vi "DFD M-Band Filter Bank Decomposition (Array).vi"(7 "init? (F)":bool, 8 "error in (no error)":errorcluster, 10 "filter bank in":T1 {"mFBank_SynthesisFilters"."mMRate_SumWl" min=1 max=32 step=1; "mFBank_SynthesisFilters"."mMRate_InputIwl" min=1 max=32 step=1; "mFBank_SynthesisFilters"."mMRate_GainWl" min=1 max=32 step=1; "mFBank_SynthesisFilters"."mMRate_OutputWl" min=1 max=32 step=1; "mFBank_SynthesisFilters"."mMRate_InputWl" min=1 max=32 step=1; "mFBank_SynthesisFilters"."mMRate_CoefWl" min=1 max=32 step=1; "mFBank_SynthesisFilters"."mMRate_Mode" items=["Default"=-1, "No Rate Change"=0, "Interpolation"=1, "Decimation"=2, "Interpolated"=3, "Rational"=4]; "mFBank_AnalysisFilters"."mMRate_SumWl" min=1 max=32 step=1; "mFBank_AnalysisFilters"."mMRate_InputIwl" min=1 max=32 step=1; "mFBank_AnalysisFilters"."mMRate_GainWl" min=1 max=32 step=1; "mFBank_AnalysisFilters"."mMRate_OutputWl" min=1 max=32 step=1; "mFBank_AnalysisFilters"."mMRate_InputWl" min=1 max=32 step=1; "mFBank_AnalysisFilters"."mMRate_CoefWl" min=1 max=32 step=1; "mFBank_AnalysisFilters"."mMRate_Mode" items=["Default"=-1, "No Rate Change"=0, "Interpolation"=1, "Decimation"=2, "Interpolated"=3, "Rational"=4]; "mFBank_Type" items=["Uniform", "Non-Uniform"]}, 11 "signal in":dbl[](array[numeric]) format="%.2f") -> (0 "error out":errorcluster, 3 "subband signals":dbl[][](array[numeric]))   [LabVIEW 2017, in "NI_DigFilter_FilterBank.lvlib"]
doc: "Decomposes a signal into M-band signals continuously with a cosine-modulated filter bank."
uses:
  <vilib>/addons/Digital Filter Design/NI_DigFilter_FilterBank.lvlib
  <vilib>/addons/Digital Filter Design/FilterBank.llb/Object/DFD Filter Bank Obj.ctl
  <vilib>/addons/Digital Filter Design/_Objects.llb/DFD Multirate Filter Obj.ctl
  <vilib>/addons/Digital Filter Design/_Objects.llb/DFD Multirate Mode.ctl
  <vilib>/addons/Digital Filter Design/_Objects.llb/DFD Coef Norm Type.ctl
  <vilib>/addons/Digital Filter Design/_Objects.llb/DFD Round-off Mode.ctl
  <vilib>/addons/Digital Filter Design/_Objects.llb/DFD FXP MRate Multiply Mode.ctl
  <vilib>/addons/Digital Filter Design/FilterBank.llb/Object/DFD Filter Bank Processing Method.ctl
  <vilib>/addons/Digital Filter Design/FilterBank.llb/Object/DFD Filter Bank Type.ctl
  <vilib>/addons/Digital Filter Design/FilterBank.llb/Process/DFD M-Band Filter Bank Decomposition with State (Array).vi
  <vilib>/addons/Digital Filter Design/NI_DigFilterLicensed.lvlib
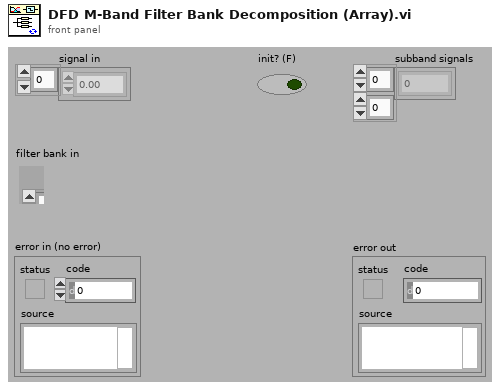
[diagram p1: front panel]
types:
  T1 = typedef "NI_DigFilter_FilterBank.lvlib/DFD Filter Bank Obj.ctl" = cluster{"mFBank_AnalysisFilters":T2[], "mFBank_SynthesisFilters":T2[], "mFBank_#Bands":i32, "mFBank_ProcMethod":T7, "mFBank_Coeffs":dbl[], "mFBank_Gain":dbl, "mFBank_Delay":i32, "mFBank_Type":T8}
  T2 = typedef "NI_DigFilterLicensed.lvlib/DFD Multirate Filter Obj.ctl" = cluster{"mMRate_Structure":enum16{"CIC", "FIR", "IIR", "Lattice"}, "mMRate_Mode":T3, "mMRate_Factor":i32, "mMRate_FIRParams":cluster{"mMRate_FIR_H":dbl[], "mMRate_FIR_IsNyquist?":bool, "mMRate_FIR_IsSymmetric?":bool}, "mMRate_CICParams":cluster{"mMRate_CIC_#Stage":i32, "mMRate_CIC_Lag":i32, "mMRate_CIC_Type":enum16{"Lowpass", "Highpass"}}, "mMRate_Order":i32, "mMRate_Version":string, "mMRate_Comments":string, "mMRate_RationalFactor":cluster{"mMRate_L":i32, "mMRate_M":i32}, "mMRate_Fs":dbl, "mMRate_Quantized?":bool, "mMRate_QFilterGain":dbl, "mMRate_CoefWl":i16, "mMRate_Scaling":cluster{"mMRate_ScaleByPowerOf2?":bool, "mMRate_ScaleType":T4}, "mMRate_InputWl":i16, "mMRate_OutputWl":i16, "mMRate_OutputMode":T5, "mMRate_MultMode":T6, "mMRate_BitPruning":bool, "mMRate_GainWl":i16, "mMRate_OutputFwl":i16, "mMRate_SumIwl":i16, "mMRate_InputIwl ":i16, "mMRate_SumWl":i16, "mMRate_CoefIwl":i16}
  T3 = typedef "NI_DigFilterLicensed.lvlib/DFD Multirate Mode.ctl" = i16
  T4 = typedef "NI_DigFilterLicensed.lvlib/DFD Coef Norm Type.ctl" = enum16{"No Norm", "Time Domain 1-Norm", "Time Domain 2-Norm", "Time Domain Inf-Norm"}
  T5 = typedef "NI_DigFilterLicensed.lvlib/DFD Round-off Mode.ctl" = enum16{"Nearest", "Truncation"}
  T6 = typedef "NI_DigFilterLicensed.lvlib/DFD FXP MRate Multiply Mode.ctl" = enum16{"Truncated", "Full"}
  T7 = typedef "NI_DigFilter_FilterBank.lvlib/DFD Filter Bank Processing Method.ctl" = enum16{"General", "2-Band QMF Lattice", "Cosine-Modulated"}
  T8 = typedef "NI_DigFilter_FilterBank.lvlib/DFD Filter Bank Type.ctl" = u16
  T9 = typedef "NI_DigFilter_FilterBank.lvlib/DFD Bank Obj.ctl" = cluster{"mBank_Filters":T2[], " mBank_#Bands":i32, "mBank_ProcMethod":T7, "mBank_Coeffs":dbl[], "mBank_Gain":dbl, "mBank_Type":T8}
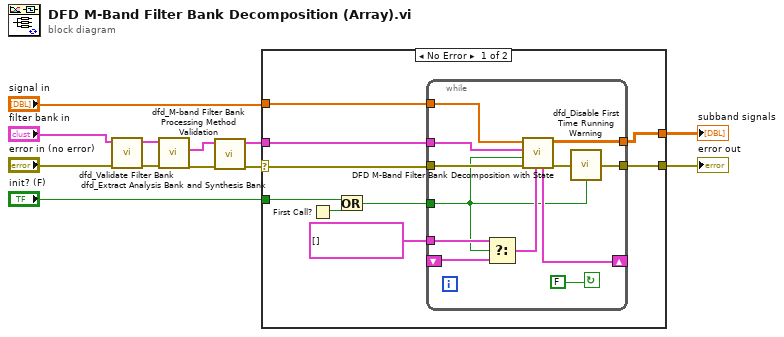
[diagram p0: block diagram]
diagram:
  n1 = call <vilib>:"dfd_Validate Filter Bank.vi"("error in (no error)"="error in (no error)", "filter banks in"="filter bank in") -> ("error out"=w7:errorcluster, "filter bank out"=w6:T1)  [unwired: 7 in, 1 out]
  n2 = call <vilib>:"dfd_Extract Analysis Bank and Synthesis Bank.vi"("error in (no error)"=w7, "filter banks in"=w6) -> ("error out"=w10:errorcluster, "analysis bank"=w9:T9)  [unwired: 6 in, 2 out]
  n3 = call <vilib>:"dfd_M-band Filter Bank Processing Method Validation.vi"("error in (no error)"=w10, "bank in"=w9) -> ("error out"=w3:errorcluster, "dup bank"=w4:T9)  [unwired: 8 in]
  n4 = case shown="No Error" w3 {
    selector: w3 -> [w18 w34]
    tunnel: "signal in" -> [w21 _]
    tunnel: [w20 w34] -> w12
    tunnel: [w19 _] -> w11
    tunnel: "init? (F)" -> [w14 _]
    tunnel: w4 -> [w17 _]
    frame No Error {
      n5 = First Call?() -> (First Call?: T/F=w16:bool)
      n6 = Or(x=w14, y=w16) -> (x .or. y?=w15:bool)
      n7 = while {
        tunnel: w17 -> [w33]
        tunnel: w18 -> [w32]
        shift-right: [w30] -> _
        shift-left: _ -> [w25]
        tunnel: w15 -> [w22]
        tunnel: cluster{"signal in":dbl[]}[] [] ("appended array") -> [w31]
        tunnel: w21 -> [w28]
        tunnel: [w23] -> w20
        tunnel: [w27] -> w19
        stop <- FALSE continue-if-true
        n8 = Select(t=w31, s=w22, f=w25) -> (s? t:f=w26:cluster{"state ":dbl[]}[])
        n9 = call-poly <vilib>:"DFD M-Band Filter Bank Decomposition with State.vi"("state in"=w26, "error in (no error)"=w32, "init?"=w22, "analysis bank"=w33, "M bands"=w28) -> ("error out"=w24:errorcluster, "y"=w27:dbl[][], "state out"=w30:cluster{"state ":dbl[]}[])  [unwired: 4 in]
        n10 = call <vilib>:"dfd_Disable First Time Running Warning.vi"("error in"=w24, "disable?"=w22) -> ("error out"=w23:errorcluster)
      }
    }
    frame Error {
    }
  }
  "error out" <- w12
  "subband signals" <- w11
